vi "DAQAnalog_Examples.vi"() -> ()   [LabVIEW 2020]
uses:
  <vilib>/DAQmx/read.llb/DAQmx Read (Analog 1D Wfm NChan NSamp).vi
  <vilib>/DAQmx/miscellaneous.llb/DAQmx Fill In Error Info.vi
panel:
  out "error out":errorcluster
  in  "DAQ Board Name":tag
  in  "Canales":tag[](array[tag])
  in  "number of samples":i32=1000
  in  "error in":errorcluster
  in  "rate":dbl=1000.0 format="%0.2f"
  out "data":waveform(dbl)[](graph)
  in  "stop":bool
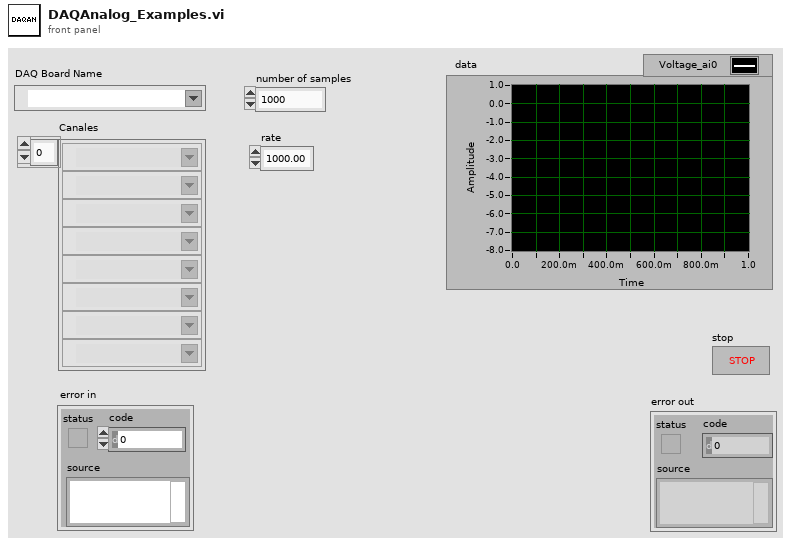
[diagram p1: front panel]
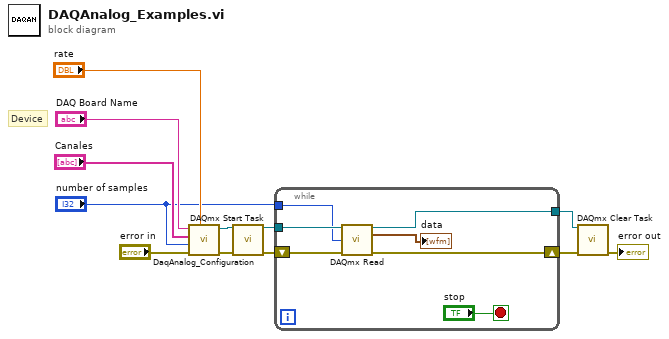
[diagram p0: block diagram]
diagram:
  # "Device"
  n1 = call "DaqAnalog_Configuration.vi"("Sampling Frequency"="rate", "error in"="error in", "Number of Samples"="number of samples", "Canales"="Canales", "DAQ Board Name"="DAQ Board Name") -> ("error out"=w7:errorcluster, "task out"=w8:refnum<k21>)  [unwired: 5 in]
  n2 = call <vilib>:"DAQmx Start Task.vi"("task/channels in"=w8, "error in"=w7) -> ("task out"=w12:refnum<k21>, "error out"=w11:errorcluster)  [unwired: 12 in]
  n3 = while {
    tunnel: w12 -> [w19]
    tunnel: [w16] -> w9
    shift-right: [w15] -> w10
    shift-left: w11 -> [w18]
    tunnel: "number of samples" -> [w13]
    stop <- "stop" stop-if-true
    n4 = call-poly <vilib>:"DAQmx Read.vi"("task/channels in"=w19, "number of samples per channel"=w13, "error in"=w18) -> ("task out"=w16:refnum<k21>, "data"=→"data":waveform(dbl)[], "error out"=w15:errorcluster)  [unwired: 10 in]
  }
  n5 = call <vilib>:"DAQmx Clear Task.vi"("task in"=w9, "error in"=w10) -> ("error out"=→"error out":errorcluster)  [unwired: 13 in]
